vi "MiniPCompareData.vi"(8 "all rows 3":dbl[][](array[numeric]), 9 "Alt Limit":string, 10 "Referans Veriler":string[](array[string]), 11 "Veri Aralığı":i32[](array[numeric])) -> (2 "all rows":dbl[][](array[numeric]), 3 "CompareXY":T1(graph))   [LabVIEW 2021]
uses:
  <vilib>/Utility/file.llb/Read Delimited Spreadsheet (DBL).vi
panel:
  in  "Grafik Sayısı":string
  in  "all rows 2":dbl[][](array[numeric])=array485x24[11640 elements]
  out "Numeric 2":i32
  out "Numeric":i32
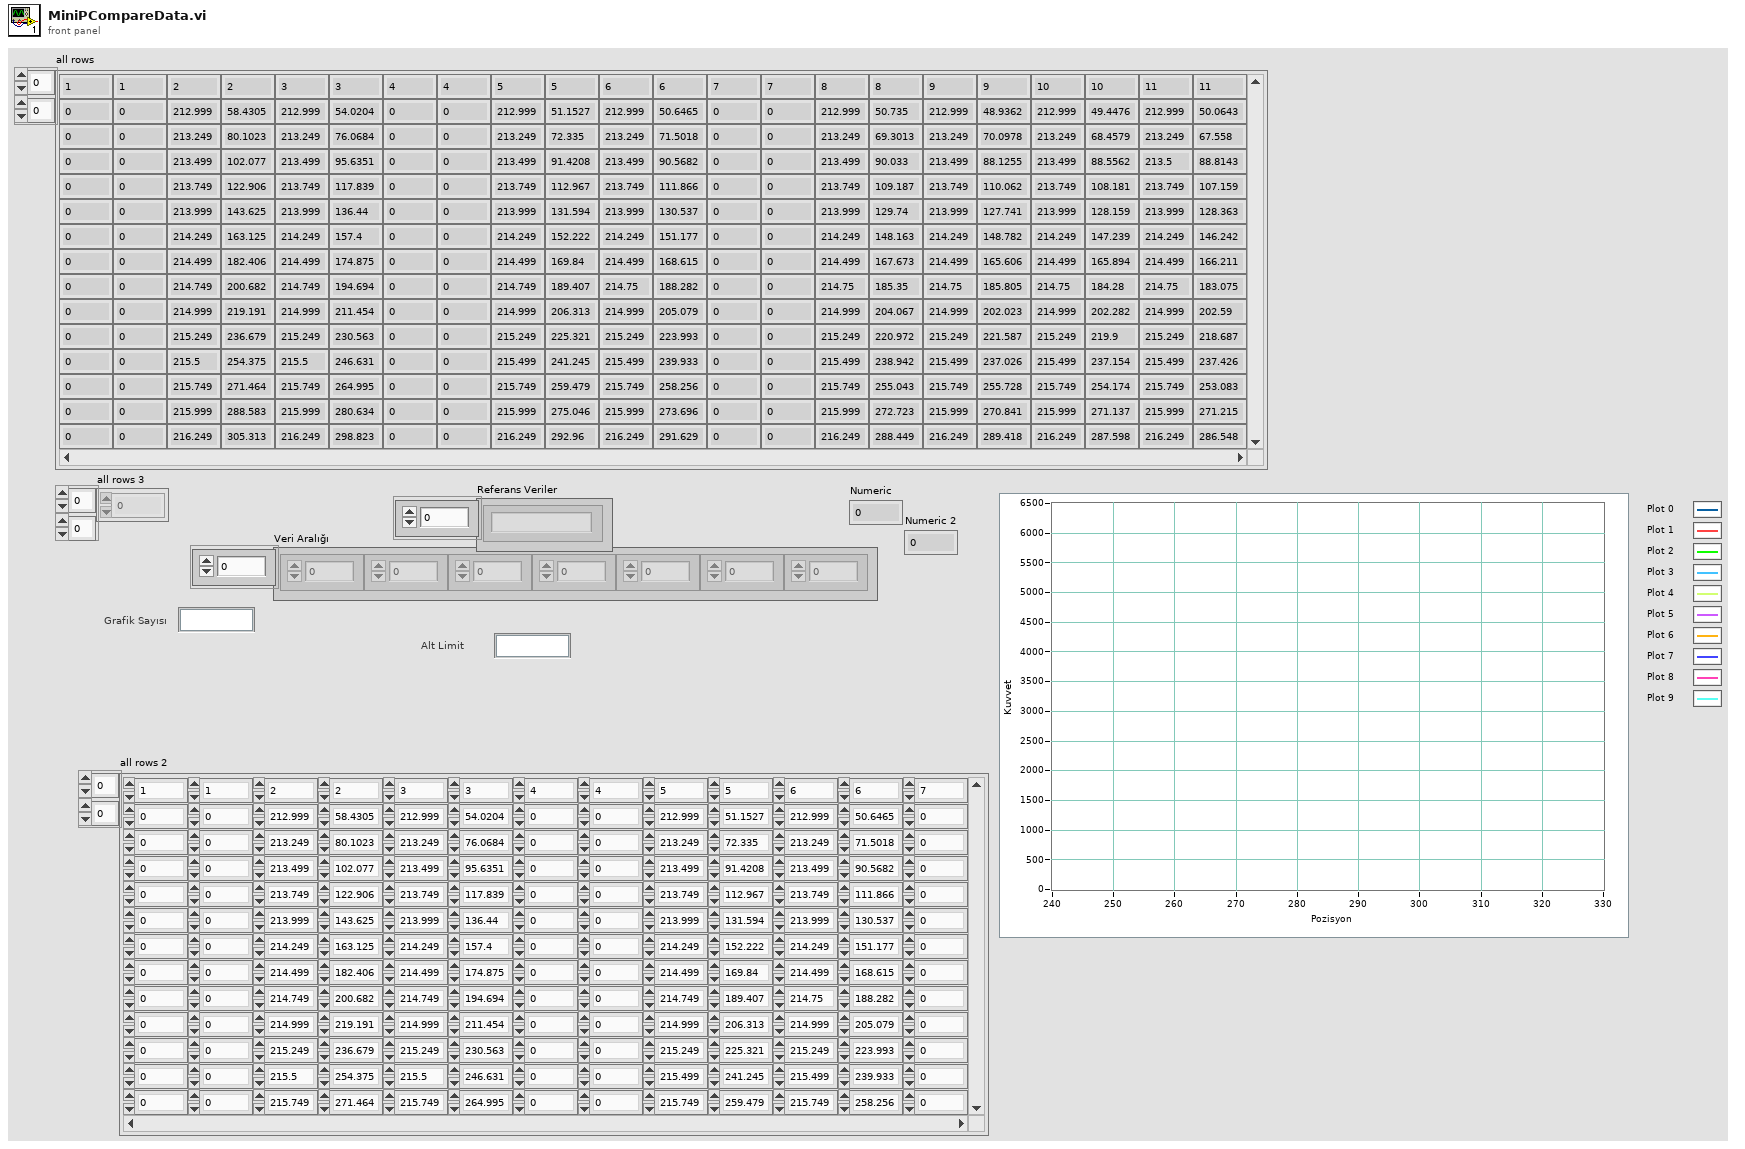
[diagram p1: front panel]
types:
  T1 = cluster{"Item Names":dbl[], "Item Names":dbl[]}[]
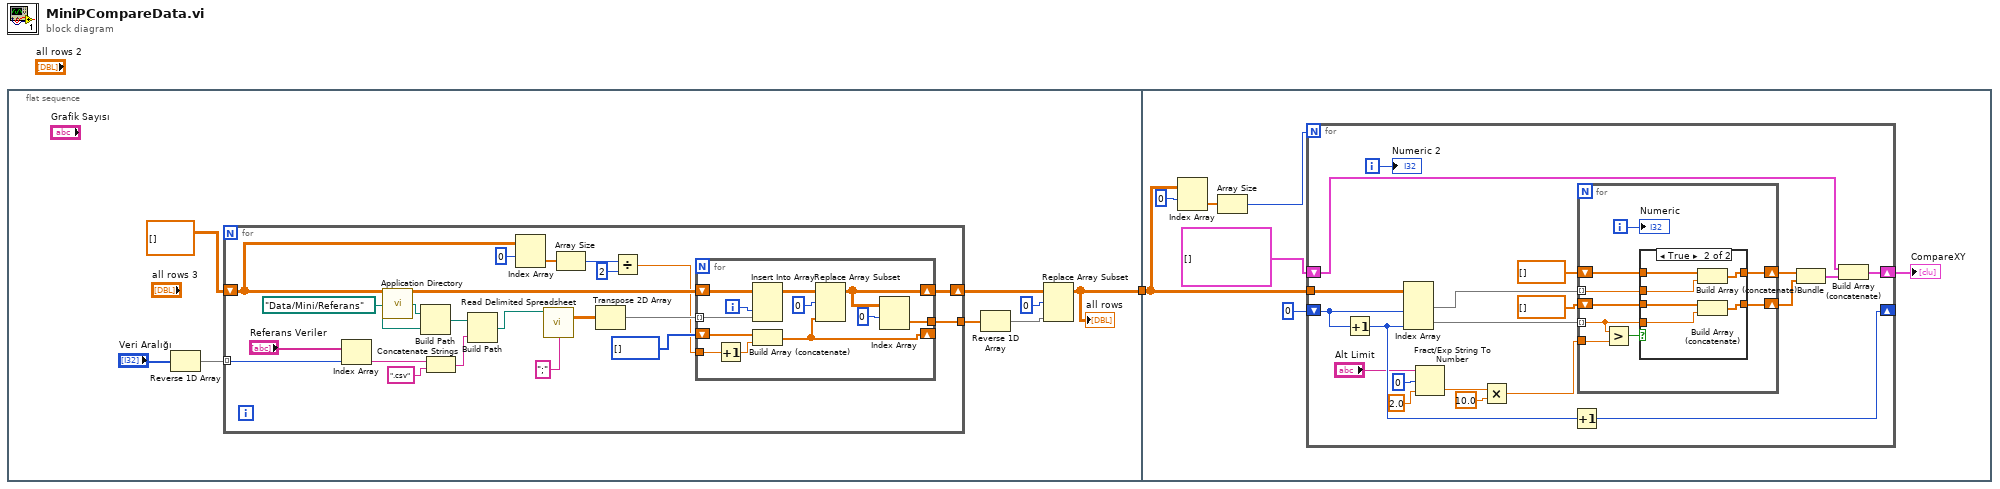
[diagram p0: block diagram]
diagram:
  n1 = flat-sequence {
    tunnel: [w3] -> w1
    tunnel: w1 -> [w44]
    frame #0 {
      n2 = Reverse 1D Array(array="Veri Aralığı") -> (reversed array=w8:i32[])
      n3 = for {
        shift-right: [w17] -> w4
        shift-left: dbl[][] [] ("all rows 3") -> [w14]
        tunnel: w8 -> [w19] mode=indexing
        tunnel: [w18] -> w6
        n4 = Index Array(array="Referans Veriler", index=w19) -> (element=w22:string)
        n5 = call <vilib>:"Application Directory.vi"() -> ("Application Directory"=w27:path)
        n6 = Build Path(base path=w27, name or relative path=path "Data/Mini/Referans") -> (appended path=w25:path)
        n7 = Concatenate Strings(w22, ".csv" ("string")) -> (w30:string)
        n8 = Build Path(base path=w25, name or relative path=w30) -> (appended path=w29:path)
        n9 = Index Array(array=w14, index (row)=0 ("index")) -> (element=w13:dbl[])  [unwired: 1 in]
        n10 = call-poly <vilib>:"Read Delimited Spreadsheet.vi"("file path (dialog if empty)"=w29, "delimiter (\\t)"=";" ("delimiter (\\t)")) -> ("all rows"=w21:dbl[][])  [unwired: 8 in, 5 out]
        n11 = Array Size(array=w13) -> (size(s)=w12:i32)
        n12 = Transpose 2D Array(2D array=w21) -> (transposed array=w20:dbl[][])
        n13 = Divide(x=w12, y=2) -> (x/y=w10:dbl)
        n14 = for {
          shift-right: [w34] -> w17
          shift-left: w14 -> [w42]
          tunnel: w20 -> [w41] mode=indexing
          shift-right: [w35] -> _
          shift-left: i32[] [] ("size(s)") -> [w40]
          tunnel: [w32] -> w18
          tunnel: w10 -> [w31]
          i -> [w38]
          n15 = Increment(x=w31) -> (x+1=w39:dbl)
          n16 = Insert Into Array(array=w42, index (col)=w38, new element=w41) -> (w37:dbl[][])  [unwired: 1 in]
          n17 = Build Array (concatenate)(w40, w39) -> (w35:dbl[])
          n18 = Replace Array Subset(array=w37, new element=w35, index (row)=0) -> (w34:dbl[][])  [unwired: 1 in]
          n19 = Index Array(array=w34, index (row)=0) -> (element=w32:dbl[])  [unwired: 1 in]
        }
      }
      n20 = Reverse 1D Array(array=w6) -> (reversed array=w7:dbl[])
      n21 = Replace Array Subset(array=w4, new element=w7, index (row)=0) -> (w3:dbl[][])  [unwired: 1 in]
      "all rows" <- w3
    }
    frame #1 {
      n22 = Index Array(array=w44, index (row)=0) -> (element=w43:dbl[])  [unwired: 1 in]
      n23 = Array Size(array=w43) -> (size(s)=w45:i32)
      n24 = for {
        N: w45 -> [_]
        tunnel: w44 -> [w50]
        shift-right: [w68] -> _
        shift-left: 0 -> [w69]
        shift-right: [w64] -> w47
        shift-left: T1 [] -> [w65]
        i -> [w55]
        n25 = Increment(x=w69) -> (x+1=w67:i32)
        n26 = Index Array(array=w50, index (col) #1=w69, index (col) #2=w67) -> (element #1=w60:dbl[], element #2=w61:dbl[])  [unwired: 2 in]
        n27 = Fract/Exp String To Number(string="Alt Limit", offset=0, default (0 dbl)=2.0 ("default (0 DBL)")) -> (number=w53:dbl)  [unwired: 1 in, 1 out]
        n28 = Multiply(x=w53, y=10.0) -> (x*y=w52:dbl)
        n29 = Increment(x=w67) -> (x+1=w68:i32)
        n30 = for {
          tunnel: w52 -> [w78]
          tunnel: w61 -> [w70] mode=indexing
          shift-right: [w76] -> w58
          shift-left: dbl[] [] -> [w77]
          tunnel: w60 -> [w71] mode=indexing
          shift-right: [w72] -> w59
          shift-left: dbl[] [] -> [w75]
          i -> [w74]
          n31 = Greater?(x=w70, y=w78) -> (0:w73:bool)
          n32 = case shown="True" w73 {
            tunnel: w77 -> [w80 w86]
            tunnel: [w80 w85] -> w76
            tunnel: w70 -> [_ w81]
            tunnel: w71 -> [_ w82]
            tunnel: w75 -> [w79 w84]
            tunnel: [w79 w83] -> w72
            frame False {
            }
            frame True {
              n33 = Build Array (concatenate)(w84, w82) -> (w83:dbl[])
              n34 = Build Array (concatenate)(w86, w81) -> (w85:dbl[])
            }
          }
          "Numeric" <- w74
        }
        n35 = Bundle(w59, w58) -> (w66:cluster{dbl[], dbl[]})  [unwired: 1 in]
        n36 = Build Array (concatenate)(w65, w66) -> (w64:T1)
        "Numeric 2" <- w55
      }
      "CompareXY" <- w47
    }
  }
